vi "IFD Tag Total Size.vi"(8 "error in (no error)":errorcluster, 10 "Add Strip":bool=TRUE, 11 "IFD in":refnum<class "IFD.lvclass">) -> (0 "error out":errorcluster, 2 "Size(byte)":u32, 3 "IFD out":refnum<class "IFD.lvclass">)   [LabVIEW 2016, in "IFD.lvclass"]
uses:
  IFD.lvclass
  IFD.lvclass/IFD.ctl
  Tag/IFD_Tag.lvclass/IFD_Tag.ctl
  Tag/IFD_Tag.lvclass
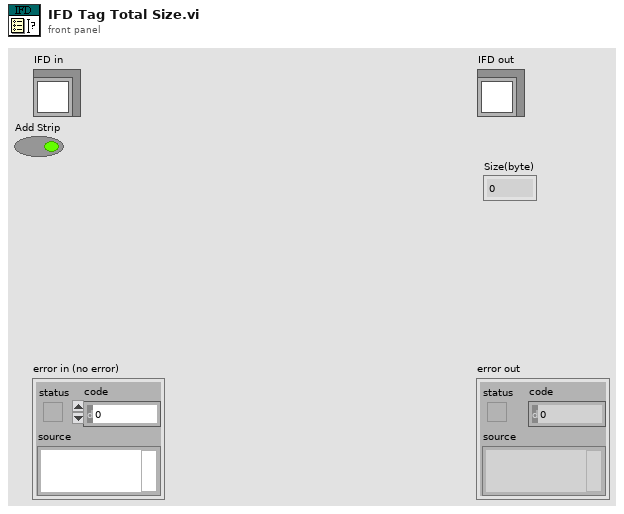
[diagram p1: front panel]
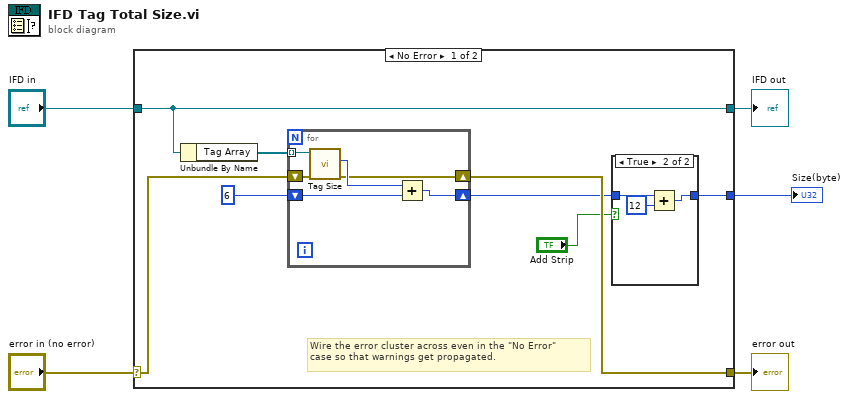
[diagram p0: block diagram]
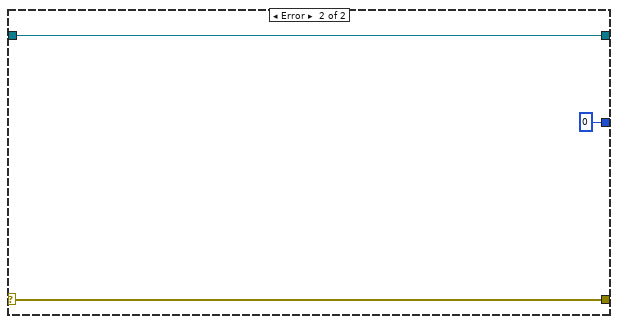
[diagram p3: hidden frame]
diagram:
  n1 = case shown="No Error" "error in (no error)" {
    selector: "error in (no error)" -> [w10 w26]
    tunnel: [w9 w26] -> w4
    tunnel: [w13 w25] -> w2
    tunnel: "IFD in" -> [w13 w25]
    tunnel: [w6 u32 0] -> w1
    frame No Error {
      # "Wire the error cluster across even in the \"No Error\"\ncase so that warnings get propagated."
      n2 = Unbundle By Name(w13) -> ("Tag Array"=w12:refnum<class "IFD_Tag.lvclass">[])
      n3 = for {
        tunnel: w12 -> [w23] mode=indexing
        shift-right: [w20] -> w7
        shift-left: u32 6 -> [w22]
        shift-right: [w18] -> w9
        shift-left: w10 -> [w19]
        n4 = call "Tag Size.vi"("error in (no error)"=w19, "IFD_Tag in"=w23) -> ("error out"=w18:errorcluster, "Byte Count"=w21:u32)  [unwired: 6 in, 2 out]
        n5 = Add(x=w21, y=w22) -> (x+y=w20:u32)
      }
      n6 = case shown="True" "Add Strip" {
        tunnel: w7 -> [w14 w17]
        tunnel: [w14 w15] -> w6
        frame False {
        }
        frame True {
          n7 = Add(x=w17, y=u32 12) -> (x+y=w15:u32)
        }
      }
    }
    frame Error {
    }
  }
  "error out" <- w4
  "IFD out" <- w2
  "Size(byte)" <- w1
